vi "Test Set Column Width.vi"(11 "Test Case In":refnum<class "Test Open Xml.lvclass">) -> (0 "error out":errorcluster, 3 "Test Case Out":refnum<class "Test Open Xml.lvclass">)   [LabVIEW 2020, in "Test Open Xml.lvclass"]
uses:
  Test Open Xml.lvclass
  C:/Program Files/National Instruments/LabVIEW 2025/vi.lib/Astemes/LUnit/Test Case.lvclass
  Source/Cell DataType.ctl
  <vilib>/Astemes/LUnit/Test Case.lvclass/Test Case.ctl
  6bd0ddee-c4a9-43dd-9f12-e32be91059bb.vi
  efeba741-6930-4178-aa8a-aa8c96a7f46d.vi
  c20d3199-2179-4aa4-a7d2-d4fd39b2aa3d.vi
  <vilib>/Astemes/LUnit/Core/LUnit Test Case/Private/Append Fail Result.vi
  <vilib>/Astemes/LUnit/Core/LUnit Test Case/Private/Append Pass Result.vi
  <vilib>/Astemes/LUnit/Core/LUnit Test Case/Private/Run In UI.vi
  <vilib>/Utility/error.llb/Clear Errors.vi
  <vilib>/Astemes/LUnit/Test Case.lvclass
  Source/Open Xml.lvlib
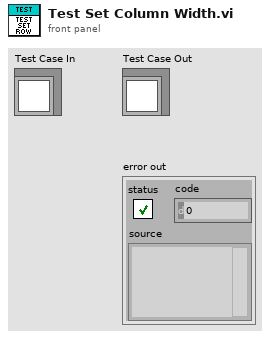
[diagram p1: front panel]
types:
  T1 = typedef "Open Xml.lvlib/Cell DataType.ctl" = enum16{"Void", "Boolean", "Number", "Error", "SharedString", "String", "InlineString", "Date"}
  T2 = cluster{"Number":dbl, "String":string, "Boolean":bool, "Time Stamp":timestamp, "Error":errorcluster}[]
  T3 = cluster{"Number":dbl, "String":string, "Boolean":bool, "Time Stamp":timestamp, "Error":errorcluster}
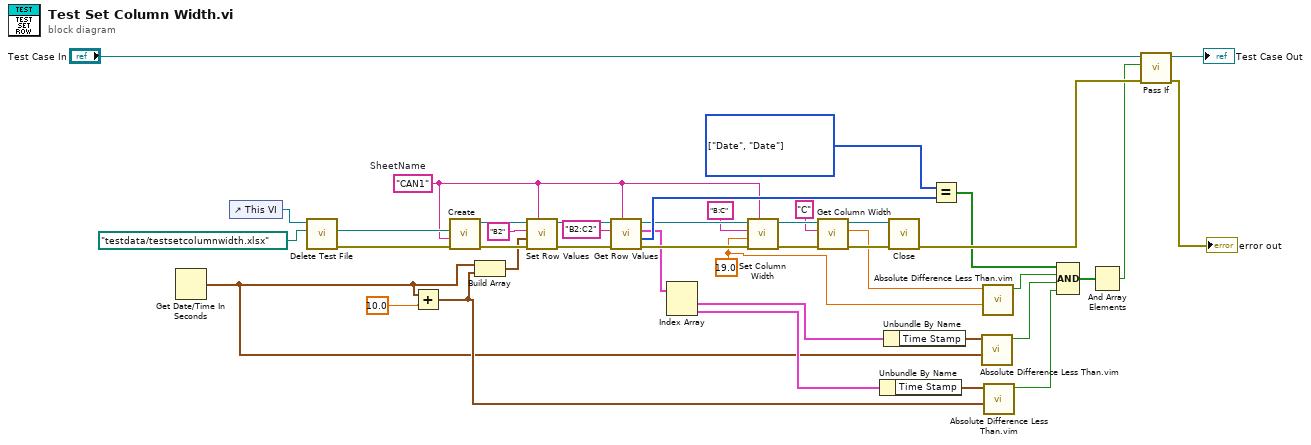
[diagram p0: block diagram]
diagram:
  w4 = 19.0 ("Width")
  w28 = T1[] [enum."Date", enum."Date"] items=["Void", "Boolean", "Number", "Error", "SharedString", "String", "InlineString", "Date"] ("x")
  w9 = "CAN1"  # SheetName
  n1 = Get Date/Time In Seconds() -> (seconds since 1Jan1904=w13:timestamp)
  n2 = control-ref of="This VI"() -> (w19:refnum<vi>)
  n3 = call "Delete Test File.vi"("name or relative path"=path "testdata/testsetcolumnwidth.xlsx", "VI in"=w19) -> ("error out"=w16:errorcluster, "deleted path"=w17:path)  [unwired: 8 in]
  n4 = Add(x=w13, y=10.0) -> (x+y=w14:timestamp)
  n5 = call "Create.vi"("error in"=w16, "SheetName"=w9, "Path"=w17) -> ("error out"=w38:errorcluster, "SpreadsheetDoc"=w39:refnum<k24>)  [unwired: 7 in]
  n6 = Build Array(w13, w14) -> (w24:timestamp[])
  n7 = call "Set Row Values.vi"("Sheet Name"=w9, "error in"=w38, "Values"=w24, "Cell Address"="B2", "SpreadsheetDoc"=w39) -> ("error out"=w34:errorcluster, "SpreadsheetDoc out"=w33:refnum<k24>)  [unwired: 5 in]
  n8 = call "Get Row Values.vi"("Sheet Name"=w9, "error in"=w34, "Row Address"="B2:C2" ("Cell Address"), "SpreadsheetDoc in"=w33) -> ("error out"=w36:errorcluster, "Types"=w32:T1[], "Cell Values"=w29:T2, "SpreadsheetDoc out"=w11:refnum<k24>)  [unwired: 4 in]
  n9 = Index Array(array=w29) -> (element #1=w27:T3, element #2=w26:T3)  [unwired: 2 in]
  n10 = call "Set Column Width.vi"("Sheet Name"=w9, "error in"=w36, "Width"=w4, "Columns Range"="B:C", "SpreadsheetDoc"=w11) -> ("error out"=w12:errorcluster, "SpreadsheetDoc out"=w7:refnum<k24>)  [unwired: 5 in]
  n11 = call "Get Column Width.vi"("error in"=w12, "Column"="C", "SpreadsheetDoc"=w7) -> ("error out"=w8:errorcluster, "Width"=w3:dbl, "SpreadsheetDoc out"=w6:refnum<k24>)  [unwired: 6 in]
  n12 = Unbundle By Name(w26) -> ("Time Stamp"=w20:timestamp)
  n13 = Unbundle By Name(w27) -> ("Time Stamp"=w21:timestamp)
  n14 = call "Close.vi"("error in"=w8, "SpreadsheetDoc"=w6) -> ("error out"=w37:errorcluster)  [unwired: 9 in]
  n15 = Equal?(x=w28, y=w32) -> (x = y?=w2:bool[])
  n16 = call "Absolute Difference Less Than.vim"("Number 2"=w13, "Number 1"=w21) -> ("In Limit"=w23:bool)  [unwired: 9 in]
  n17 = call "Absolute Difference Less Than.vim"("Number 2"=w4, "Number 1"=w3) -> ("In Limit"=w1:bool)  [unwired: 9 in]
  n18 = call "Absolute Difference Less Than.vim"("Number 2"=w14, "Number 1"=w20) -> ("In Limit"=w22:bool)  [unwired: 9 in]
  n19 = Compound Arithmetic op=AND(w2, w1, w23, w22) -> (w25:bool[])
  n20 = And Array Elements(Boolean array=w25) -> (logical AND=w35:bool)
  n21 = call <vilib>:"Pass If.vi"("error in (no error)"=w37, "Pass?"=w35, "LUnit Test Case In"="Test Case In") -> ("error out"=→"error out":errorcluster, "LUnit Test Case Out"=→"Test Case Out":refnum<class "Test Open Xml.lvclass">)  [unwired: 7 in]
